vi "Pixy_COM-RIO.vi"() -> (0 "Height":i32, 1 "Width":i32, 2 "Y":i32, 3 "X":i32, 4 "Read error out":errorcluster)   [LabVIEW 2016]
uses:
  <vilib>/Analysis/baseanly.llb/Mean (DBL).vi
  <vilib>/Instr/_visa.llb/VISA Configure Serial Port (Instr).vi
  Cam H.vi
  Cam W.vi
  Cam Y.vi
  Cam X.vi
  <vilib>/Analysis/NI_AALBase.lvlib
panel:
  in  "Command 2":string(combo)="go"
  out "Data out":T1
  out "Initialization error out":errorcluster
  out "Area":dbl(graph)
  in  "Display buffer size":u16=100 min=1
  out "Data display":string
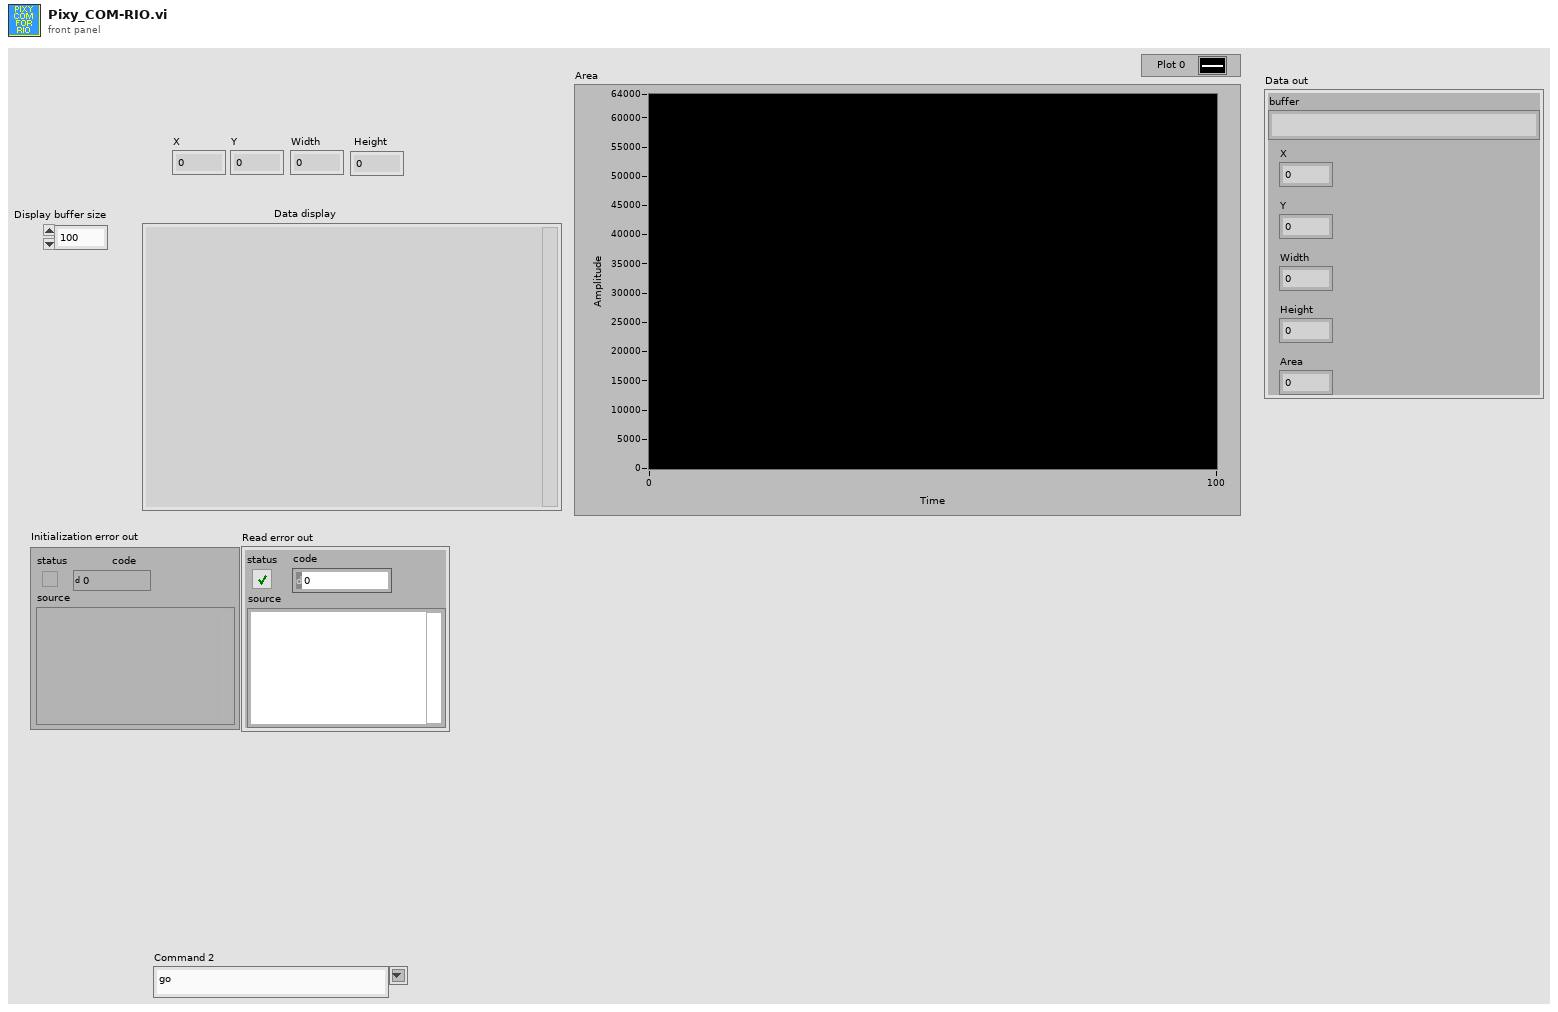
[diagram p1: front panel]
types:
  T1 = cluster{"buffer":string, "X":i32, "Y":i32, "Width":i32, "Height":i32, "Area":dbl}
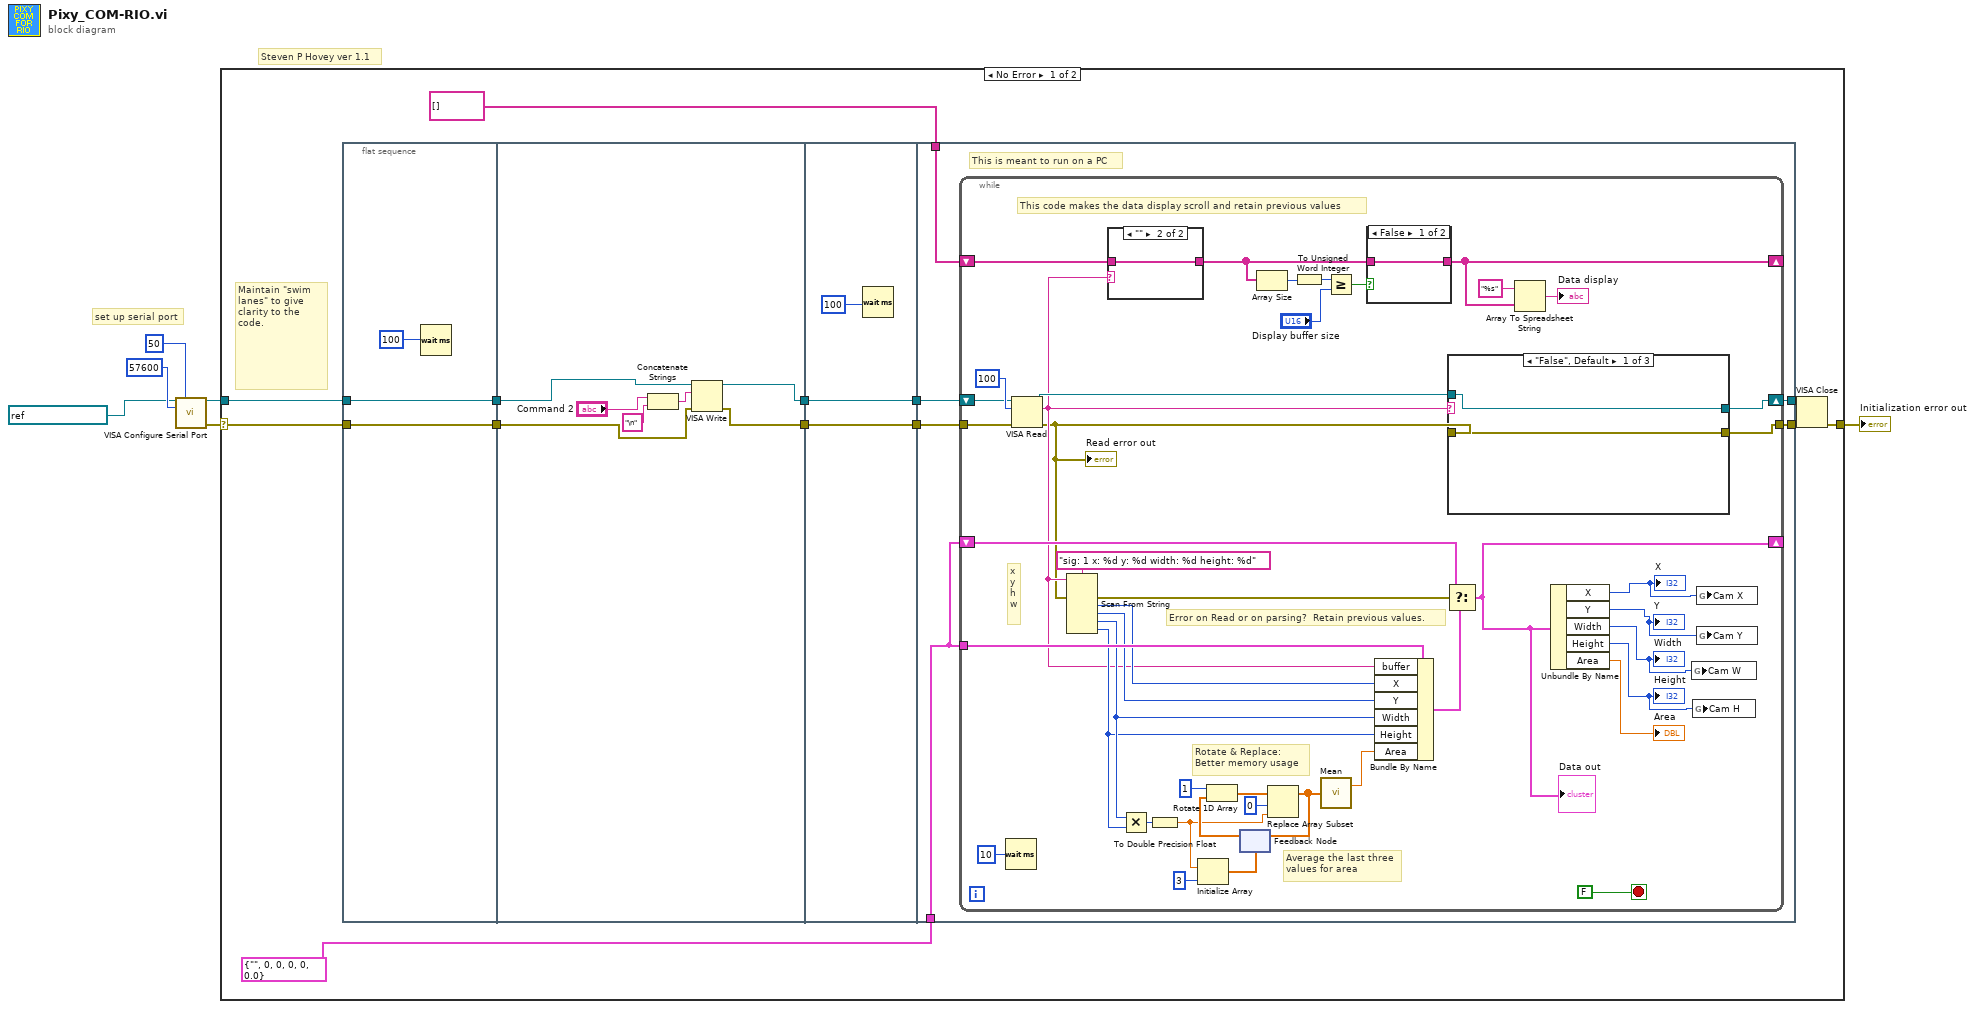
[diagram p0: block diagram]
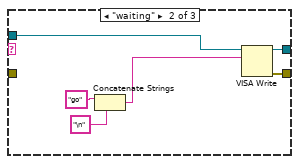
[diagram p2: hidden frame]
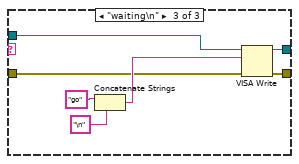
[diagram p3: hidden frame]
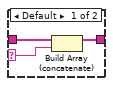
[diagram p4: hidden frame]
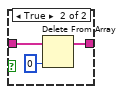
[diagram p5: hidden frame]
diagram:
  # "Steven P Hovey ver 1.1"
  # "set up serial port"
  n1 = call-poly "VISA Configure Serial Port"("VISA resource name"=refnum<visa-resource-name> "ASRL3::INSTR", "timeout (10sec)"=u32 50, "baud rate (9600)"=u32 57600) -> ("VISA resource name out"=w4:refnum<visa-resource-name>, "error out"=w2:errorcluster)  [unwired: 11 in]
  n2 = case shown="No Error" w2 {
    selector: w2 -> [w15 w106]
    tunnel: w4 -> [w19 _]
    tunnel: [w16 w106] -> w3
    frame No Error {
      # "Maintain \"swim lanes\" to give clarity to the code."
      n3 = flat-sequence {
        tunnel: w15 -> [w21]
        tunnel: w19 -> [w22]
        tunnel: [w22] -> w8
        tunnel: [w21] -> w7
        tunnel: [w25] -> w10
        tunnel: [w24] -> w9
        tunnel: w8 -> [w26]
        tunnel: w7 -> [w23]
        tunnel: [w32] -> w14
        tunnel: [w31] -> w13
        tunnel: w10 -> [w32]
        tunnel: w9 -> [w31]
        tunnel: [w37] -> w18
        tunnel: [w36] -> w17
        tunnel: w14 -> [w38]
        tunnel: w13 -> [w35]
        tunnel: T1 {"buffer"="", "X"=0, "Y"=0, "Width"=0, "Height"=0, "Area"=0.0} -> [w34]
        tunnel: string[] [] -> [w33]
        frame #0 {
          n4 = Wait (ms)(milliseconds to wait=100) -> ()  [unwired: 1 out]
        }
        frame #1 {
          n5 = Concatenate Strings("Command 2", "\n") -> (w29:string)
          n6 = VISA Write(VISA resource name=w26, write buffer=w29, error in (no error)=w23) -> (VISA resource name out=w25:refnum<visa-resource-name>, error out=w24:errorcluster)  [unwired: 1 out]
        }
        frame #2 {
          n7 = Wait (ms)(milliseconds to wait=100) -> ()  [unwired: 1 out]
        }
        frame #3 {
          # "This is meant to run on a PC"
          n8 = while {
            shift-right: [w39] -> w37
            shift-left: w38 -> [w79]
            shift-right: [w57] -> _
            shift-left: w34 -> [w59]
            shift-right: [w51] -> _
            shift-left: w33 -> [w72]
            tunnel: w34 -> [w82]
            tunnel: w35 -> [w50]
            tunnel: [w40] -> w36
            stop <- FALSE ("stop") stop-if-true
            # "Error on Read or on parsing?  Retain previous values."
            # "Rotate & Replace:\nBetter memory usage"
            # "Average the last three\nvalues for area"
            # "This code makes the data display scroll and retain previous values"
            # "x\ny\nh\nw"
            n9 = Wait (ms)(milliseconds to wait=u32 10) -> ()  [unwired: 1 out]
            n10 = VISA Read(VISA resource name=w79, byte count=u32 100, error in (no error)=w50) -> (VISA resource name out=w43:refnum<visa-resource-name>, read buffer=w42:string, error out=w41:errorcluster)  [unwired: 1 out]
            "Read error out" <- w41
            n11 = Scan From String(format string="sig: 1 x: %d y: %d width: %d height: %d", input string=w42, error in=w41) -> (error out=w60:errorcluster, output 1=w65:i32, output 2=w64:i32, output 3=w63:i32, output 4=w62:i32)  [unwired: 5 in, 2 out]
            n12 = case shown="\"\"" w42 {
              selector: w42 -> [w98 _]
              tunnel: w72 -> [w99 w101]
              tunnel: [w100 w101] -> w52
              frame Default {
                n13 = Build Array (concatenate)(w99, w98) -> (w100:string[])
              }
              frame "" {
              }
            }
            n14 = Multiply(x=w63, y=w62) -> (x*y=w61:i32)
            n15 = To Double Precision Float(number=w61) -> (double precision float=w53:dbl)
            n16 = Initialize Array(w53, 3 ("dimension size")) -> (w76:dbl[])
            n17 = feedback #1(w76) -> (w56:dbl[])
            n18 = Rotate 1D Array(1:w56, 2:1 ("n")) -> (0:w55:dbl[])
            n19 = Array Size(array=w52) -> (size(s)=w70:i32)
            n20 = Replace Array Subset(array=w55, new element=w53, index=0) -> (w75:dbl[])
            n21 = feedback-in #1(w75) -> ()
            n22 = To Unsigned Word Integer(number=w70) -> (unsigned 16bit integer=w69:u16)
            n23 = call-poly <vilib>:"Mean.vi"("X"=w75) -> ("mean"=w78:dbl)  [unwired: 1 out]
            n24 = Greater Or Equal?(x=w69, y="Display buffer size") -> (x >= y?=w68:bool)
            n25 = case shown="False" w68 {
              tunnel: w52 -> [w102 w105]
              tunnel: [w102 w104] -> w51
              frame False {
              }
              frame True {
                n26 = Delete From Array(array=w105, index=0) -> (array with subset deleted=w104:string[])  [unwired: 1 in, 1 out]
              }
            }
            n27 = Bundle By Name(cluster=w82, "buffer"=w42, "X"=w65, "Y"=w64, "Width"=w63, "Height"=w62, "Area"=w78) -> (w58:T1)
            n28 = Select(t=w59, s=w60, f=w58) -> (s? t:f=w57:T1)
            "Data out" <- w57
            n29 = case shown="\"False\", Default" w42 {
              tunnel: w43 -> [w84 w90 w97]
              tunnel: [w84 w89 w96] -> w39
              tunnel: [w83 w88 w95] -> w40
              tunnel: w41 -> [w83 _ w91]
              frame "False", Default {
              }
              frame "waiting" {
                n30 = Concatenate Strings("go", "\n") -> (w85:string)
                n31 = VISA Write(VISA resource name=w90, write buffer=w85) -> (VISA resource name out=w89:refnum<visa-resource-name>, error out=w88:errorcluster)  [unwired: 1 in, 1 out]
              }
              frame "waiting\n" {
                n32 = Concatenate Strings("go", "\n") -> (w92:string)
                n33 = VISA Write(VISA resource name=w97, write buffer=w92, error in (no error)=w91) -> (VISA resource name out=w96:refnum<visa-resource-name>, error out=w95:errorcluster)  [unwired: 1 out]
              }
            }
            n34 = Array To Spreadsheet String(array=w51, 3:"%s" ("format string")) -> (spreadsheet string=→"Data display":string)  [unwired: 1 in]
            n35 = Unbundle By Name(w57) -> ("X"=w45:i32, "Y"=w44:i32, "Width"=w47:i32, "Height"=w46:i32, "Area"=→"Area":dbl)
            "X" <- w45
            "Y" <- w44
            "Width" <- w47
            "Height" <- w46
            n36 = global write "Cam W.vi" "Cam W"(w47) -> ()
            n37 = global write "Cam H.vi" "Cam H"(w46) -> ()
            n38 = global write "Cam X.vi" "Cam X"(w45) -> ()
            n39 = global write "Cam Y.vi" "Cam Y"(w44) -> ()
          }
        }
      }
      n40 = VISA Close(VISA resource name=w18, error in (no error)=w17) -> (error out=w16:errorcluster)
    }
    frame Error {
    }
  }
  "Initialization error out" <- w3
